vi "Initialize Stream.vi"(8 "error in (no error)":errorcluster, 11 "Channel GUI in":refnum<class "Channel GEI.lvclass">) -> (0 "error out":errorcluster, 3 "Channel GUI out":refnum<class "Channel GEI.lvclass">)   [LabVIEW 2018, in "Channel GEI.lvclass"]
uses:
  Channel GEI.lvclass
  Channel GEI.lvclass/Channel GEI.ctl
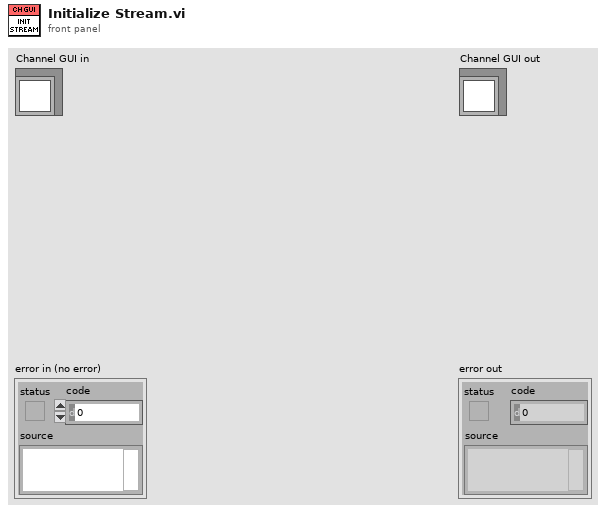
[diagram p1: front panel]
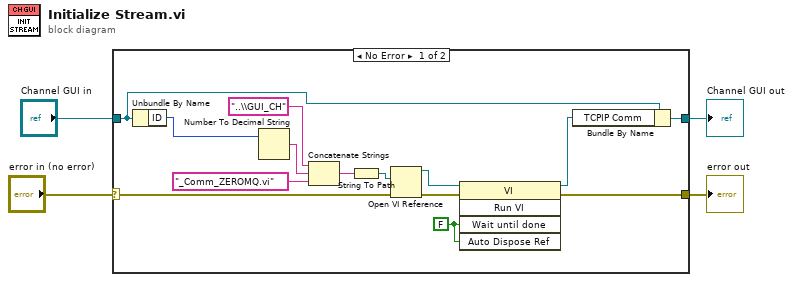
[diagram p0: block diagram]
diagram:
  n1 = case shown="No Error" "error in (no error)" {
    selector: "error in (no error)" -> [w6 w20]
    tunnel: [w7 w20] -> w4
    tunnel: [w14 w19] -> w3
    tunnel: "Channel GUI in" -> [w15 w19]
    frame No Error {
      w17 = FALSE ("Wait Until Done")
      n2 = Unbundle By Name(w15) -> ("ID"=w12:u8)
      n3 = Number To Decimal String(number=w12) -> (decimal integer string=w8:string)  [unwired: 1 in]
      n4 = Concatenate Strings("..\\GUI_CH" ("name or relative path"), w8, "_Comm_ZEROMQ.vi" ("name or relative path")) -> (w10:string)
      n5 = String To Path(string=w10) -> (path=w11:path)
      n6 = Open VI Reference(vi path=w11, error in (no error)=w6) -> (vi reference=w18:refnum<vi>, error out=w13:errorcluster)  [unwired: 4 in]
      n7 = invoke class="VI" method="Run VI"(reference=w18, error in=w13, "Wait until done"=w17, "Auto Dispose Ref"=w17) -> (reference out=w9:refnum<vi>, error out=w7:errorcluster)  [unwired: 1 in, 3 out]
      n8 = Bundle By Name(cluster=w15, "TCPIP Comm"=w9) -> (w14:refnum<class "Channel GEI.lvclass">)
    }
    frame Error {
    }
  }
  "error out" <- w4
  "Channel GUI out" <- w3
